vi "CSM - Build Exit Messages of CSMs.vi"(0 "State With Arguments (\"Macro: Exit“)":string="Macro: Exit", 7 "CSMs":string[](array[string])) -> (4 "States":string)   [LabVIEW 2017, in "Communicable State Machine.lvlib"]
doc: "Concatenates and generates exit messages (\"Macro: Exit\") based on input CSM module names.\n\n\n\n-- <b>Controls</b> --\n\n- <b>CSMs</b>: Array of CSM module names.\n- <b>State with Arguments(\"Macro: Exit\")</b>: Exit message.\n\n-- <b>Indicators</b> --\n\n- <b>States</b>: The concatenated generated CSM message string."
uses:
  Communicable State Machine.lvlib
  _Polymophic/Build Synchronous Message with Arguments.vi
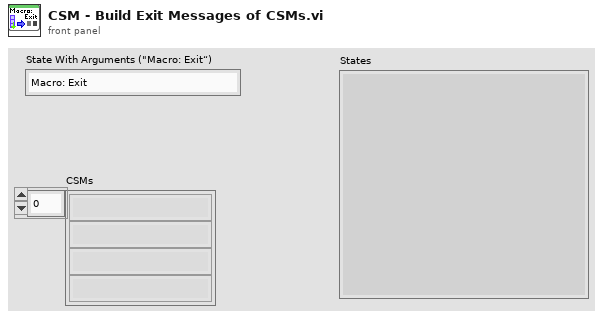
[diagram p1: front panel]
types:
  T1 = typedef "Communicable State Machine.lvlib/_CSM_MODE.ctl" = enum16{"Not Exist", "Stand Alone", "CSM", "Worker", "Worker Agent", "Chain Node", "Chain"}
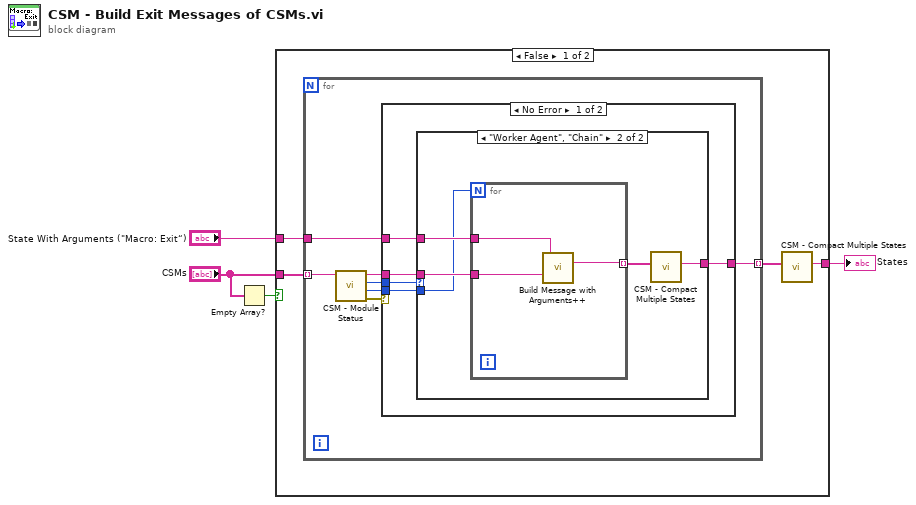
[diagram p0: block diagram]
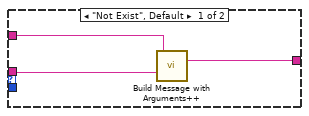
[diagram p2: hidden frame]
diagram:
  n1 = Empty Array?(array="CSMs") -> (empty?=w1:bool)
  n2 = case shown="False" w1 {
    tunnel: [w7 _] -> w4
    tunnel: "State With Arguments (\"Macro: Exit“)" -> [w6 _]
    tunnel: "CSMs" -> [w5 _]
    frame False {
      n3 = for {
        tunnel: w5 -> [w15] mode=indexing
        tunnel: [w12] -> w8 mode=indexing
        tunnel: w6 -> [w9]
        n4 = call "CSM - Module Status.vi"("CSM Name"=w15) -> ("error out"=w11:errorcluster, "#Nodes"=w13:i32, "Mode"=w10:T1, "CSM Name (Dup)"=w14:string)  [unwired: 6 in, 1 out]
        n5 = case shown="No Error" w11 {
          tunnel: w14 -> [w20 _]
          tunnel: w9 -> [w19 _]
          tunnel: w13 -> [w18 _]
          tunnel: [w17 _] -> w12
          tunnel: w10 -> [w16 _]
          frame No Error {
            n6 = case shown="\"Worker Agent\", \"Chain\"" w16 {
              tunnel: w20 -> [w22 w28]
              tunnel: w19 -> [w21 w27]
              tunnel: w18 -> [_ w26]
              tunnel: [w23 w24] -> w17
              frame "Not Exist", Default {
                n7 = call-poly "Build Message with Arguments++.vi"("State With Arguments"=w21, "Target Module (\"\")"=w22) -> ("CSM Message String"=w23:string)  [unwired: 13 in]
              }
              frame "Worker Agent", "Chain" {
                n8 = for {
                  N: w26 -> [_]
                  tunnel: w28 -> [w31]
                  tunnel: w27 -> [w30]
                  tunnel: [w29] -> w25 mode=indexing
                  n9 = call-poly "Build Message with Arguments++.vi"("State With Arguments"=w30, "Target Module (\"\")"=w31) -> ("CSM Message String"=w29:string)  [unwired: 13 in]
                }
                n10 = call "CSM - Compact Multiple States.vi"("Multiple States"=w25) -> ("States"=w24:string)  [unwired: 9 in]
              }
            }
          }
          frame Error {
          }
        }
      }
      n11 = call "CSM - Compact Multiple States.vi"("Multiple States"=w8) -> ("States"=w7:string)  [unwired: 9 in]
    }
    frame True {
    }
  }
  "States" <- w4
